vi "Scripting_ConvertNativeSubClassToBaseClass.vi"(0 "SubClass":refnum<vi>, 1 "Create/Init-VI name":string="_Init[.]vi", 2 "Destroy/CleanUp-VI name":string="CleanUp[.]vi", 5 "error in (no error)":errorcluster) -> (19 "error out":errorcluster)   [LabVIEW 2020]
uses:
  <resource>/Framework/Providers/Open_GDS/ClassProviders/Provider_LvNativeClass/Templates/LvNativeTemplateNames.ctl
  <resource>/Framework/Providers/Open_GDS/ClassProviders/Provider_LvNativeClass/ClassWriterNative_class/ClassWriterNative.lvclass
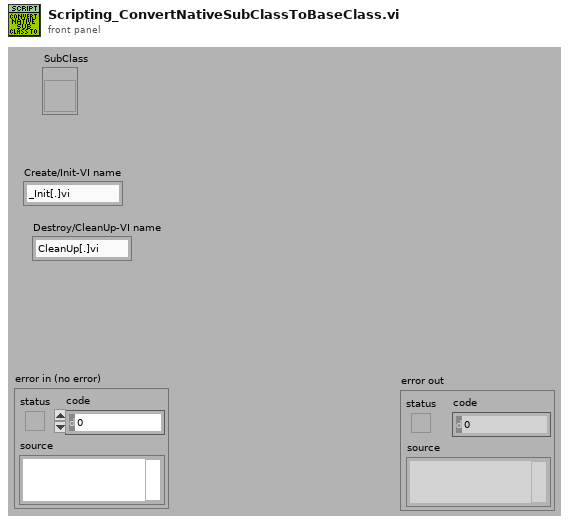
[diagram p1: front panel]
types:
  T1 = cluster{"SubCreate ":path, "ThisSubClass":refnum<vi>, "CurrentBaseClass":refnum<vi>, "SubDestroy":path, "BaseCreate ":path, "BaseDestroy":path, "ThisSubClassName":string, "AllSubClassFiles":path[], "AppRef":refnum<vi>}
  T2 = typedef "LvNativeTemplateNames.ctl" = enum16{"NativeBaseTemplate", "NativeSubTemplate", "NativeBaseTemplate_4x4x4", "NativeSubTemplate_4x4x4"}
  T3 = typedef "GDSLvCLass_ClassSettingsType.ctl" = cluster{"ClassProviderName":string, "ClassTemplateUsed":string, "ClassTemplateVersion":string, "ClassDescription":string, "PlugIns":T4[], "ConnectorPanePattern":string}
  T4 = typedef "GDSLvClass_PlugIn.ctl" = cluster{"Type":T5, "ID":string, "Version":string, "Path":path, "Name":string, "Data":variant}
  T5 = typedef "GDSLvClass_PlugInTypes.ctl" = enum16{"DesignPattern", "MethodTypes"}
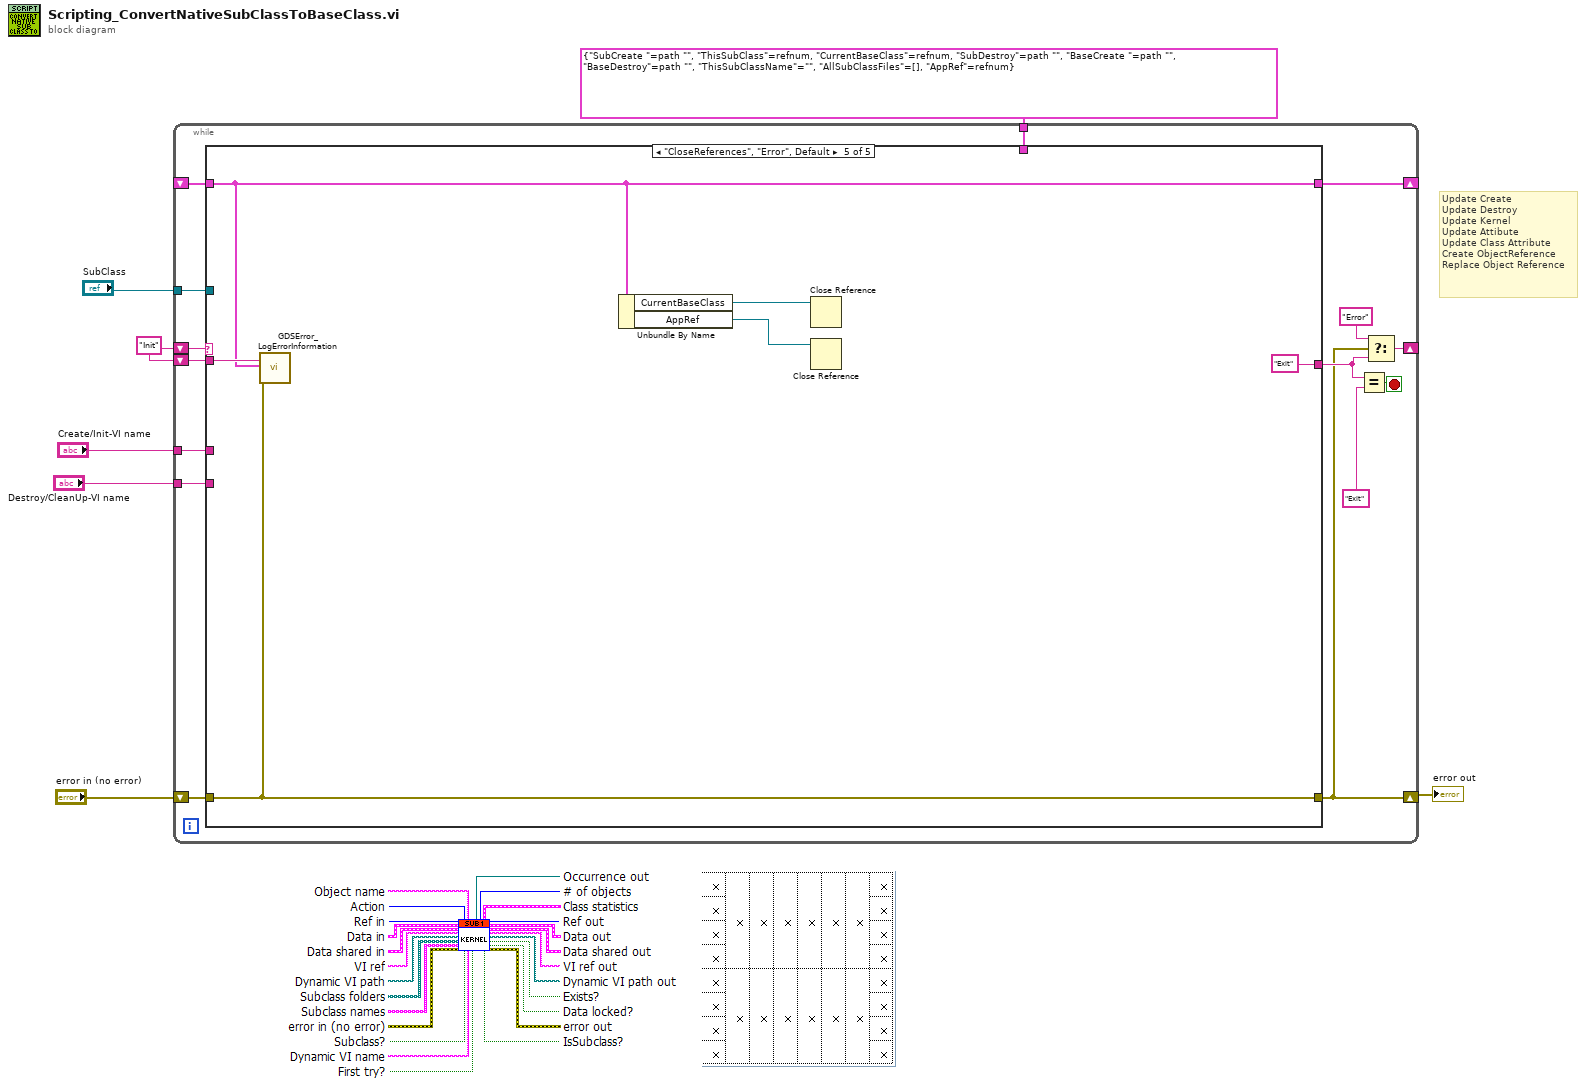
[diagram p0: block diagram]
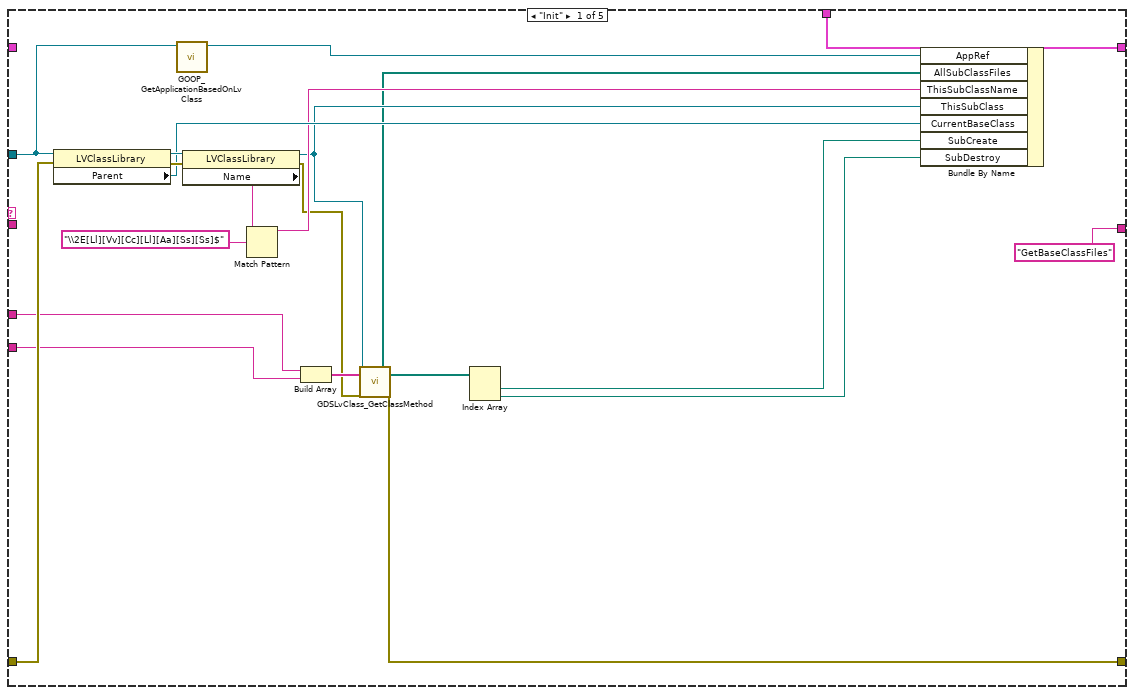
[diagram p2: hidden frame]
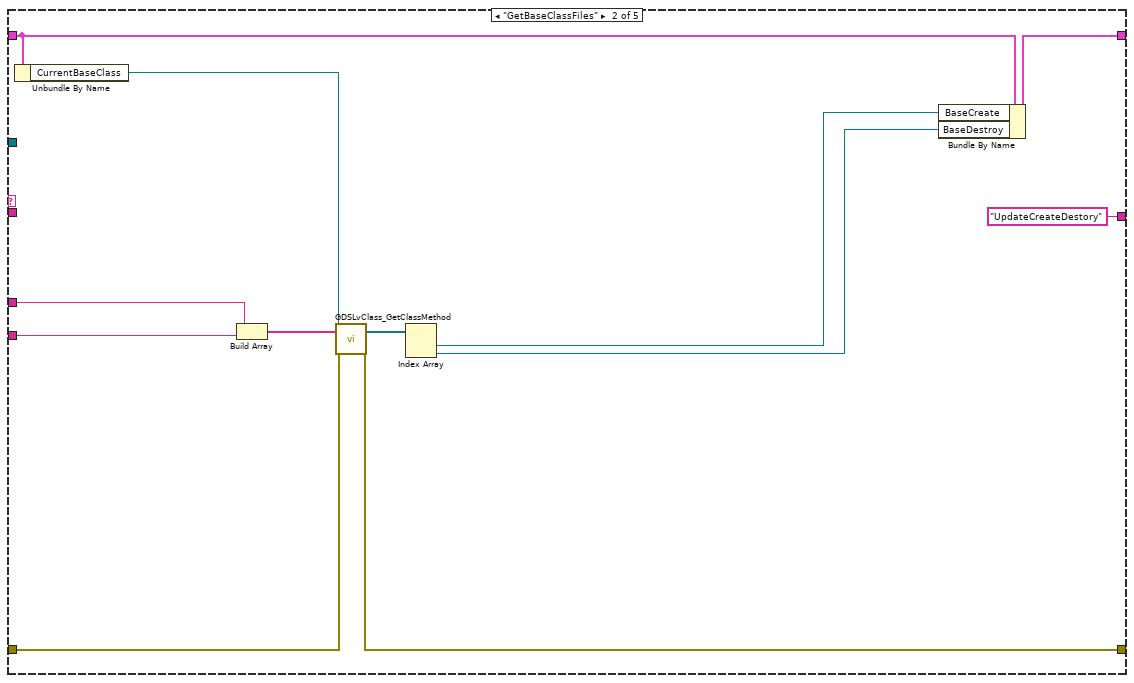
[diagram p3: hidden frame]
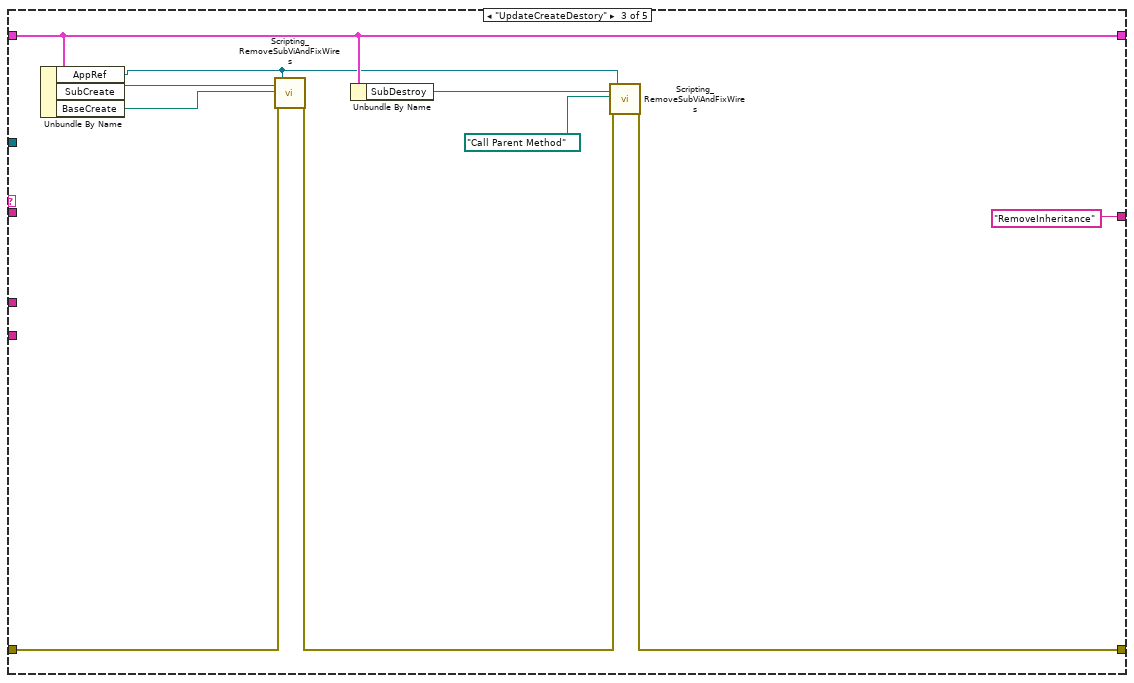
[diagram p4: hidden frame]
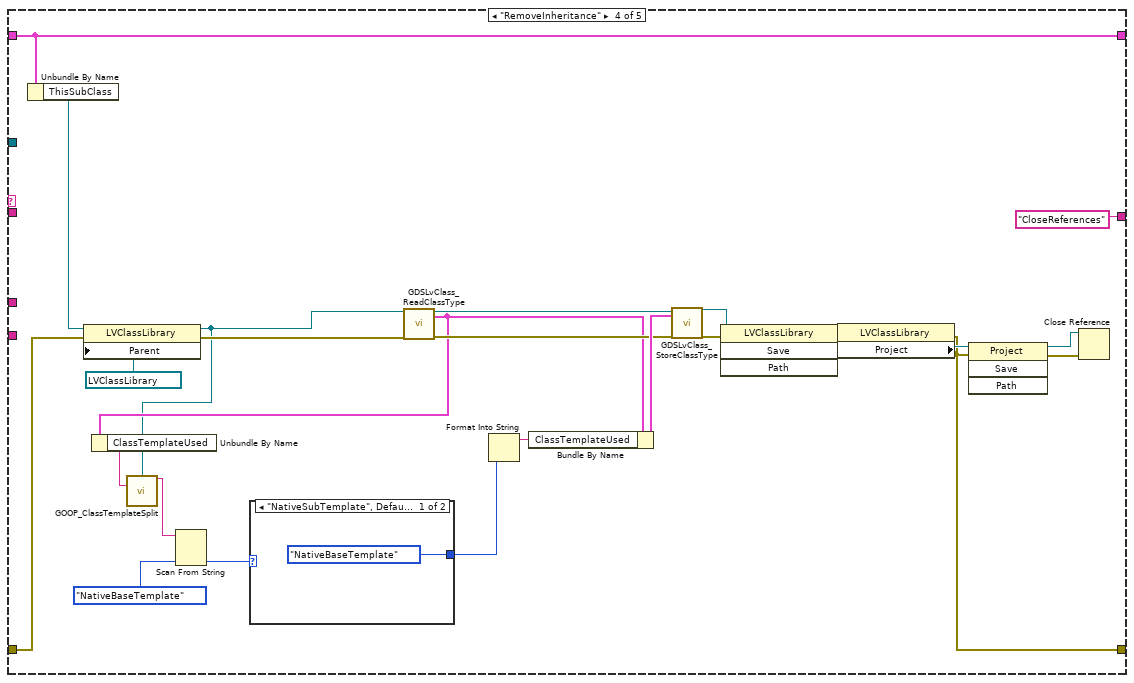
[diagram p5: hidden frame]
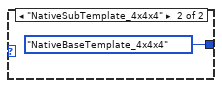
[diagram p6: hidden frame]
diagram:
  w3 = "Init"
  # "Update Create\nUpdate Destroy\nUpdate Kernel\nUpdate Attibute\nUpdate Class Attribute\nCreate ObjectReference\nReplace Object Reference"
  n1 = while {
    shift-right: [w15] -> w6
    shift-left: "error in (no error)" -> [w22]
    shift-right: [w20] -> _
    shift-left: w3 -> [w21]
    shift-right: [w14] -> _
    shift-left: _ -> [w13]
    tunnel: "SubClass" -> [w12]
    tunnel: T1 {"SubCreate "=path "", "ThisSubClass"=refnum, "CurrentBaseClass"=refnum, "SubDestroy"=path "", "BaseCreate "=path "", "BaseDestroy"=path "", "ThisSubClassName"="", "AllSubClassFiles"=[], "AppRef"=refnum} -> [w11]
    shift-left: w3 -> [w10]
    tunnel: "Create/Init-VI name" -> [w9]
    tunnel: "Destroy/CleanUp-VI name" -> [w8]
    stop <- w19 stop-if-true
    n2 = case shown="\"CloseReferences\", \"Error\", Default" w21 {
      tunnel: w22 -> [w39 w46 w63 w83 w95]
      tunnel: [w28 w45 w59 w70 w95] -> w15
      tunnel: ["GetBaseClassFiles" "UpdateCreateDestory" "RemoveInheritance" "CloseReferences" "Exit"] -> w16
      tunnel: [w43 w55 w62 w90 w96] -> w14
      tunnel: w13 -> [_ w54 w62 w90 w96]
      tunnel: w12 -> [w24 _ _ _ _]
      tunnel: w11 -> [w38 _ _ _ _]
      tunnel: w10 -> [_ _ _ _ w97]
      tunnel: w9 -> [w34 w51 _ _ _]
      tunnel: w8 -> [w33 w50 _ _ _]
      frame "Init" {
        n3 = property class="LVClassLibrary"(reference=w24, error in=w39) -> (reference out=w42:refnum<vi>, error out=w41:errorcluster, "Parent"=w40:refnum<vi>)
        n4 = call <resource>:"GOOP_GetApplicationBasedOnLvClass.vi"("LVClassLibrary in"=w24) -> ("Application out"=w23:refnum<vi>)  [unwired: 9 in, 1 out]
        n5 = property class="LVClassLibrary"(reference=w42, error in=w41) -> (reference out=w31:refnum<vi>, error out=w27:errorcluster, "Name"=w37:string)
        n6 = Match Pattern(string=w37, regular expression="\\2E[Ll][Vv][Cc][Ll][Aa][Ss][Ss]$") -> (before substring=w35:string)  [unwired: 1 in, 3 out]
        n7 = Build Array(w34, w33) -> (w32:string[])
        n8 = call <resource>:"GDSLvClass_GetClassMethod.vi"("Class Refnum In"=w31, "VINames"=w32, "error in (no error)"=w27) -> ("AllClassFiles"=w25:path[], "ViPaths"=w26:path[], "error out"=w28:errorcluster)  [unwired: 13 in, 1 out]
        n9 = Index Array(array=w26) -> (element #1=w30:path, element #2=w29:path)  [unwired: 2 in]
        n10 = Bundle By Name(cluster=w38, "AppRef"=w23, "AllSubClassFiles"=w25, "ThisSubClassName"=w35, "ThisSubClass"=w31, "CurrentBaseClass"=w40, "SubCreate"=w30, "SubDestroy"=w29) -> (w43:T1)
      }
      frame "GetBaseClassFiles" {
        n11 = Unbundle By Name(w54) -> ("CurrentBaseClass"=w47:refnum<vi>)
        n12 = Build Array(w51, w50) -> (w53:string[])
        n13 = call <resource>:"GDSLvClass_GetClassMethod.vi"("Class Refnum In"=w47, "VINames"=w53, "error in (no error)"=w46) -> ("ViPaths"=w52:path[], "error out"=w45:errorcluster)  [unwired: 13 in, 2 out]
        n14 = Index Array(array=w52) -> (element #1=w49:path, element #2=w48:path)  [unwired: 2 in]
        n15 = Bundle By Name(cluster=w54, "BaseCreate"=w49, "BaseDestroy"=w48) -> (w55:T1)
      }
      frame "UpdateCreateDestory" {
        n16 = Unbundle By Name(w62) -> ("AppRef"=w57:refnum<vi>, "SubCreate"=w65:path, "BaseCreate"=w64:path)
        n17 = call <resource>:"Scripting_RemoveSubViAndFixWires.vi"("MainViPath/ViRef/BlockDiagramRef"=w65, "SubVIToRemove"=w64, "error in (no error)"=w63, "AppRef"=w57) -> ("error out"=w60:errorcluster)  [unwired: 15 in]
        n18 = Unbundle By Name(w62) -> ("SubDestroy"=w61:path)
        n19 = call <resource>:"Scripting_RemoveSubViAndFixWires.vi"("MainViPath/ViRef/BlockDiagramRef"=w61, "SubVIToRemove"=path "Call Parent Method", "error in (no error)"=w60, "AppRef"=w57) -> ("error out"=w59:errorcluster)  [unwired: 15 in]
      }
      frame "RemoveInheritance" {
        n20 = Unbundle By Name(w90) -> ("ThisSubClass"=w84:refnum<vi>)
        n21 = property class="LVClassLibrary"(reference=w84, error in=w83, "Parent"=refnum<vi> refnum ("Parent Class")) -> (reference out=w67:refnum<vi>, error out=w77:errorcluster)
        n22 = call <resource>:"GDSLvClass_ReadClassType.vi"("Class Refnum In"=w67, "error in (no error)"=w77) -> ("Class Refnum Out"=w79:refnum<vi>, "ClassSettings"=w72:T3, "error out"=w78:errorcluster)  [unwired: 15 in]
        n23 = Unbundle By Name(w72) -> ("ClassTemplateUsed"=w68:string)
        n24 = call <resource>:"GOOP_ClassTemplateSplit.vi"("ClassItemRefIn"=w67, "FullClassTemplate"=w68) -> ("StandardTemplate"=w69:string)  [unwired: 12 in, 1 out]
        n25 = Scan From String(input string=w69, default 1=LvNativeTemplateNames."NativeBaseTemplate" ("TemplateNames")) -> (output 1=w73:T2)  [unwired: 3 in, 3 out]
        n26 = case shown="\"NativeSubTemplate\", Default" w73 {
          tunnel: [LvNativeTemplateNames."NativeBaseTemplate" ("TemplateNames") LvNativeTemplateNames."NativeBaseTemplate_4x4x4" ("TemplateNames")] -> w71
          frame "NativeSubTemplate", Default {
          }
          frame "NativeSubTemplate_4x4x4" {
          }
        }
        n27 = Format Into String(w71) -> (resulting string=w80:string)  [unwired: 3 in, 1 out]
        n28 = Bundle By Name(cluster=w72, "ClassTemplateUsed"=w80) -> (w81:T3)
        n29 = call <resource>:"GDSLvClass_StoreClassType.vi"("Class Refnum In"=w79, "ClassSettings"=w81, "error in (no error)"=w78) -> ("Class Refnum Out"=w75:refnum<vi>, "error out"=w76:errorcluster)  [unwired: 15 in]
        n30 = invoke class="LVClassLibrary" method="Save"(reference=w75, error in=w76) -> (reference out=w87:refnum<vi>, error out=w86:errorcluster)  [unwired: 2 in, 2 out]
        n31 = property class="LVClassLibrary"(reference=w87, error in=w86) -> (error out=w70:errorcluster, "Project"=w85:refnum<vi>)  [unwired: 1 out]
        n32 = invoke class="Project" method="Save"(reference=w85, error in=w70) -> (reference out=w88:refnum<vi>, error out=w89:errorcluster)  [unwired: 2 in, 2 out]
        n33 = Close Reference(reference=w88, error in (no error)=w89) -> ()  [unwired: 1 out]
      }
      frame "CloseReferences", "Error", Default {
        n34 = call <resource>:"GDSError_LogErrorInformation.vi"("State"=w97, "LocalVariableData"=w96, "error in (no error)"=w95) -> ()  [unwired: 16 in, 1 out]
        n35 = Unbundle By Name(w96) -> ("CurrentBaseClass"=w99:refnum<vi>, "AppRef"=w94:refnum<vi>)
        n36 = Close Reference(reference=w99) -> ()  [unwired: 1 in, 1 out]
        n37 = Close Reference(reference=w94) -> ()  [unwired: 1 in, 1 out]
      }
    }
    n38 = Equal?(x=w16, y="Exit") -> (x = y?=w19:bool)
    n39 = Select(t="Error", s=w15, f=w16) -> (s? t:f=w20:string)
  }
  "error out" <- w6
